vi "Record Missing Parameter.vi"(5 "Parameter":string, 7 "Found?":bool, 10 "Missing Parameters in":variant) -> (2 "Missing Parameters out":variant)   [LabVIEW 2017, in "Request.lvclass"]
uses:
  Request.lvclass
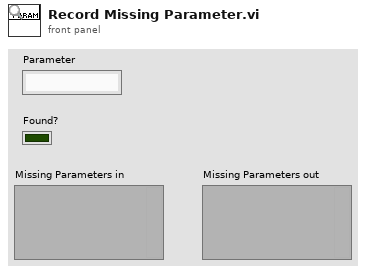
[diagram p1: front panel]
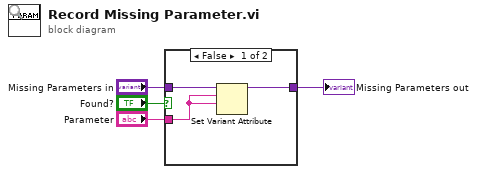
[diagram p0: block diagram]
diagram:
  n1 = case shown="False" "Found?" {
    tunnel: [w5 w8] -> w3
    tunnel: "Missing Parameters in" -> [w7 w8]
    tunnel: "Parameter" -> [w6 _]
    frame False {
      n2 = Set Variant Attribute(Variant=w7, name=w6, value=w6) -> (Variant out=w5:variant)  [unwired: 1 in, 2 out]
    }
    frame True {
    }
  }
  "Missing Parameters out" <- w3
